vi "Init UI.vi"(8 "error in (no error)":errorcluster, 11 "Configuration Window in":refnum<class "Configuration Window.lvclass">) -> (0 "error out":errorcluster, 3 "Configuration Window out":refnum<class "Configuration Window.lvclass">)   [LabVIEW 2018, in "Configuration Window.lvlib" / "Configuration Window.lvclass"]
uses:
  Configuration Window.lvclass
  Configuration Window.lvclass/Configuration Window.ctl
  <userlib>/_OpenG.lib/file/file.llb/Strip Path Extension - 1D Array of Strings__ogtk.vi
  Main Panel/LF2R IDE/LF2R IDE.lvclass
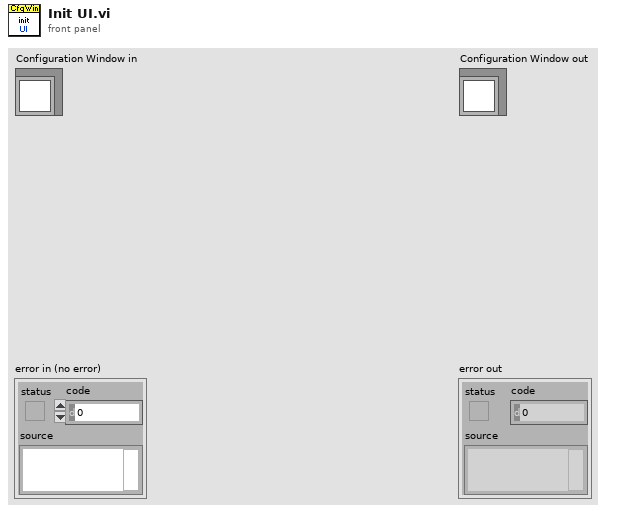
[diagram p1: front panel]
types:
  T1 = cluster{"Size":refnum<vi>, "Color":refnum<vi>, "Enable":refnum<vi>}
  T2 = cluster{"Fill Color":refnum<vi>, "Border Color":refnum<vi>, "Enable":refnum<vi>}
  T3 = cluster{"Fill Color":u32, "Border Color":u32, "Show?":bool}
  T4 = cluster{"_res_data":refnum<vi>, "_res_pngs":refnum<vi>}
  T5 = typedef "LF2R IDE.lvlib/LF2R IDE.lvclass/Const Path Setting.ctl" = cluster{"Data Folder Path":path, "PNG Folder Path":path}
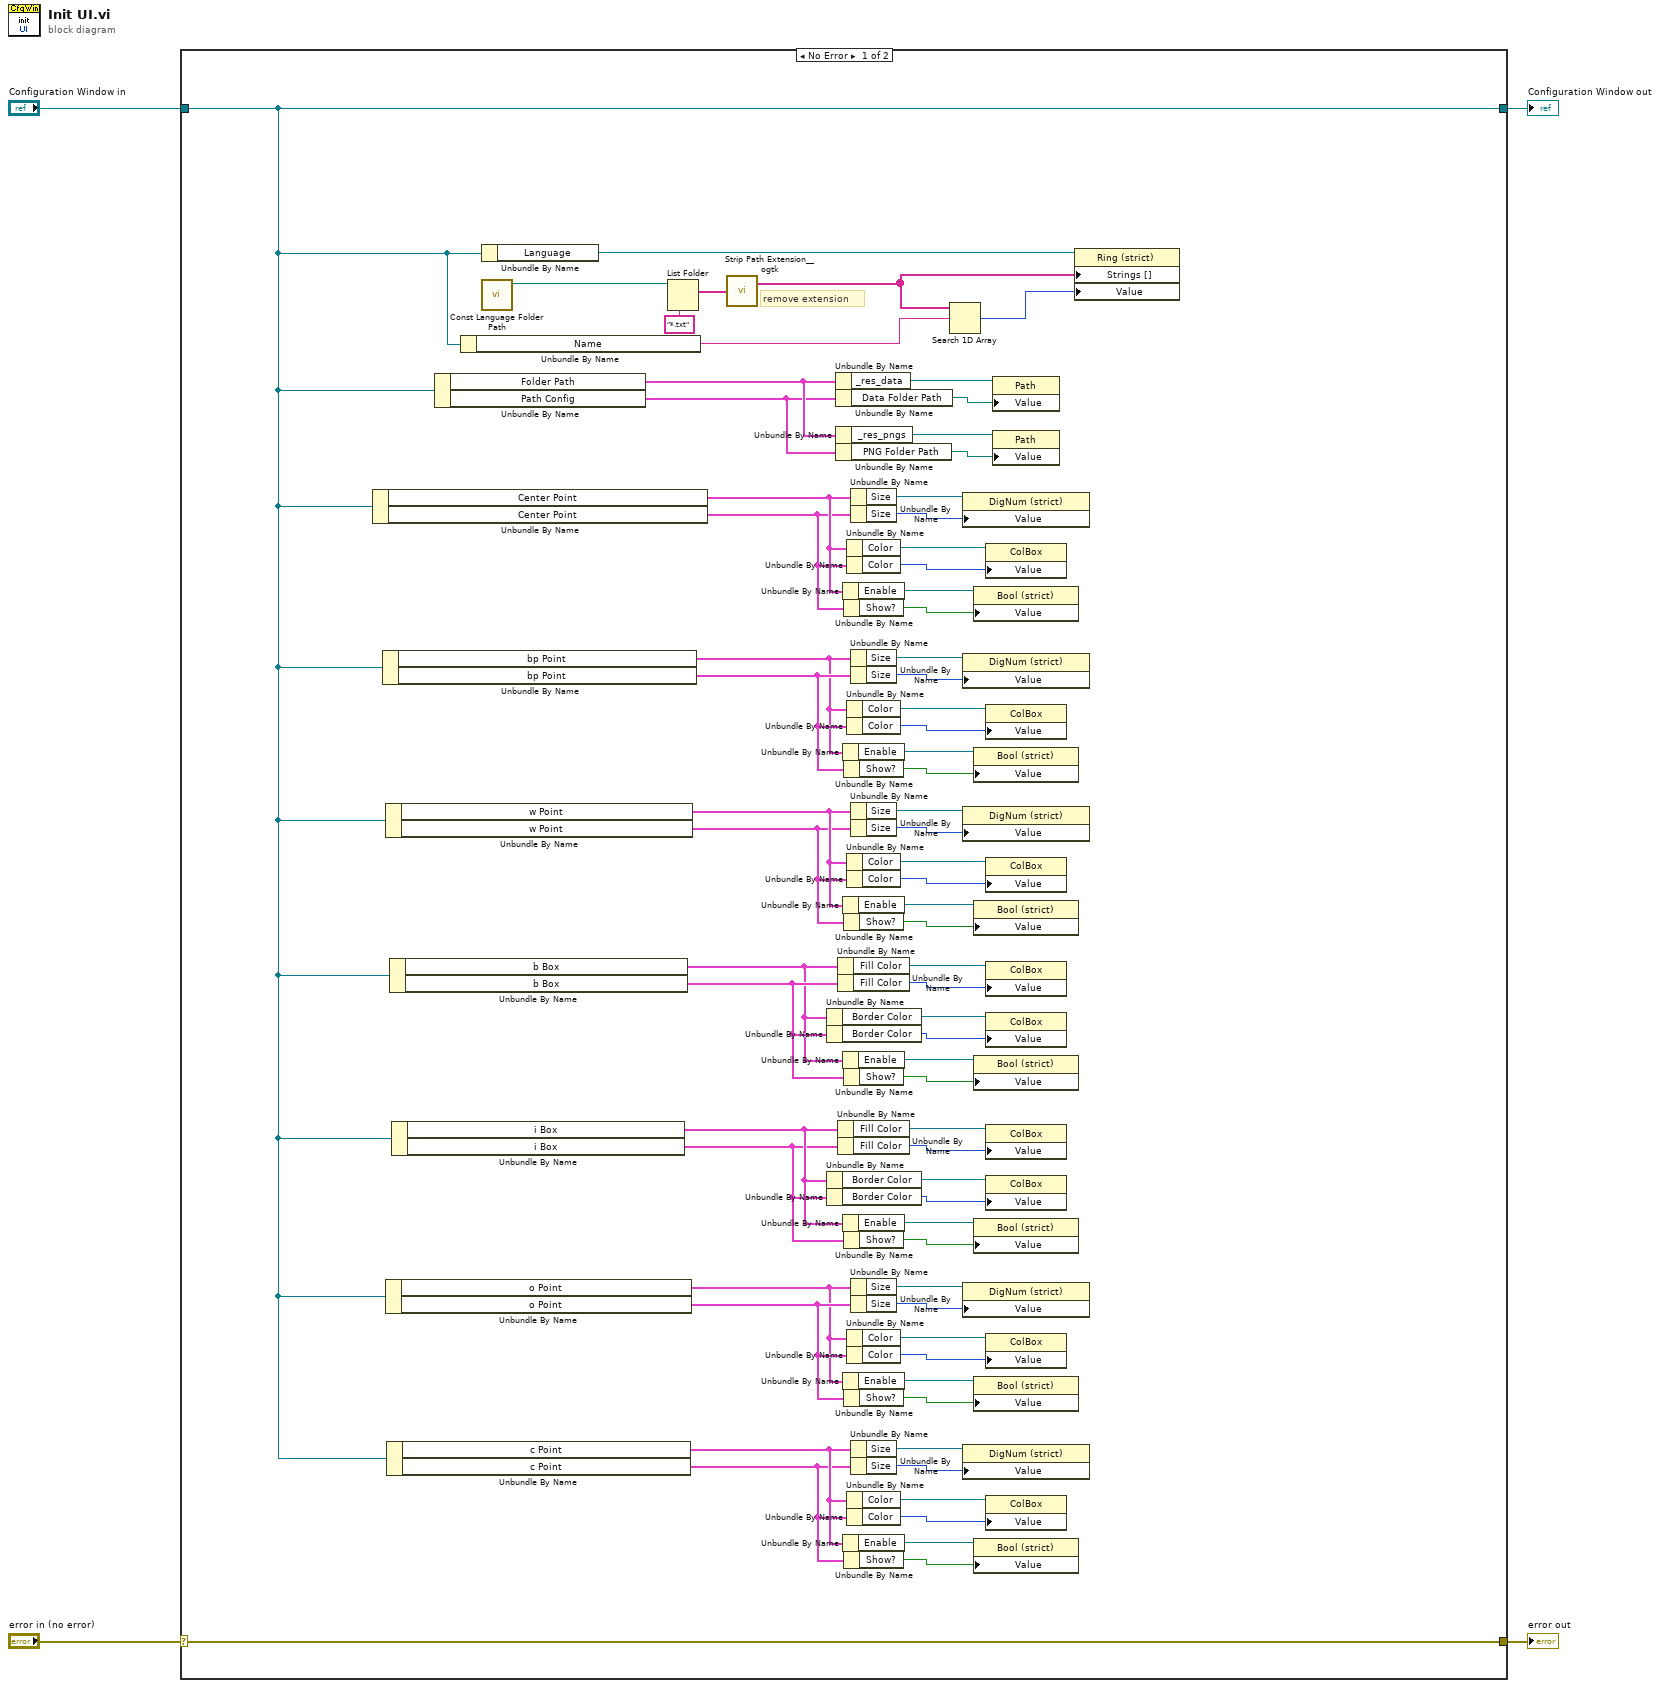
[diagram p0: block diagram]
diagram:
  n1 = case shown="No Error" "error in (no error)" {
    selector: "error in (no error)" -> [w75 w77]
    tunnel: [w75 w77] -> w3
    tunnel: [w6 w76] -> w1
    tunnel: "Configuration Window in" -> [w6 w76]
    frame No Error {
      # "remove extension"
      n2 = Unbundle By Name(w6) -> ("Center Point"=w62:T1, "Center Point"=w61:cluster{"Size":i32, "Color":u32, "Show?":bool})
      n3 = Unbundle By Name(w6) -> ("bp Point"=w59:T1, "bp Point"=w60:cluster{"Size":i32, "Color":u32, "Show?":bool})
      n4 = Unbundle By Name(w6) -> ("w Point"=w46:T1, "w Point"=w45:cluster{"Size":i32, "Color":u32, "Show?":bool})
      n5 = Unbundle By Name(w6) -> ("o Point"=w27:T1, "o Point"=w28:cluster{"Size":i32, "Color":u32, "Show?":bool})
      n6 = Unbundle By Name(w6) -> ("c Point"=w14:T1, "c Point"=w13:cluster{"Size":i32, "Color":u32, "Show?":bool})
      n7 = Unbundle By Name(w6) -> ("b Box"=w43:T2, "b Box"=w44:T3)
      n8 = Unbundle By Name(w6) -> ("i Box"=w30:T2, "i Box"=w29:T3)
      n9 = Unbundle By Name(w6) -> ("Folder Path"=w70:T4, "Path Config"=w69:T5)
      n10 = Unbundle By Name(w6) -> ("Name"=w5:string)
      n11 = Unbundle By Name(w6) -> ("Language"=w12:refnum<vi>)
      n12 = call "Const Language Folder Path.vi"() -> ("Language Folder Path"=w11:path)  [unwired: 11 in]
      n13 = List Folder(path=w11, pattern="*.txt") -> (filenames=w9:string[])  [unwired: 2 in, 3 out]
      n14 = call-poly <userlib>:"Strip Path Extension__ogtk.vi"("paths"=w9) -> ("roots"=w7:string[])  [unwired: 1 out]
      n15 = Unbundle By Name(w43) -> ("Border Color"=w40:refnum<vi>)
      n16 = Unbundle By Name(w44) -> ("Border Color"=w39:u32)
      n17 = Unbundle By Name(w30) -> ("Border Color"=w33:refnum<vi>)
      n18 = Unbundle By Name(w29) -> ("Border Color"=w34:u32)
      n19 = Unbundle By Name(w70) -> ("_res_data"=w74:refnum<vi>)
      n20 = Unbundle By Name(w69) -> ("Data Folder Path"=w73:path)
      n21 = Unbundle By Name(w70) -> ("_res_pngs"=w71:refnum<vi>)
      n22 = Unbundle By Name(w69) -> ("PNG Folder Path"=w72:path)
      n23 = Unbundle By Name(w43) -> ("Fill Color"=w37:refnum<vi>)
      n24 = Unbundle By Name(w44) -> ("Fill Color"=w38:u32)
      n25 = Unbundle By Name(w30) -> ("Fill Color"=w36:refnum<vi>)
      n26 = Unbundle By Name(w29) -> ("Fill Color"=w35:u32)
      n27 = Unbundle By Name(w62) -> ("Enable"=w64:refnum<vi>)
      n28 = Unbundle By Name(w59) -> ("Enable"=w57:refnum<vi>)
      n29 = Unbundle By Name(w46) -> ("Enable"=w48:refnum<vi>)
      n30 = Unbundle By Name(w43) -> ("Enable"=w41:refnum<vi>)
      n31 = Unbundle By Name(w30) -> ("Enable"=w32:refnum<vi>)
      n32 = Unbundle By Name(w27) -> ("Enable"=w25:refnum<vi>)
      n33 = Unbundle By Name(w14) -> ("Enable"=w16:refnum<vi>)
      n34 = Unbundle By Name(w61) -> ("Show?"=w63:bool)
      n35 = Unbundle By Name(w60) -> ("Show?"=w58:bool)
      n36 = Unbundle By Name(w45) -> ("Show?"=w47:bool)
      n37 = Unbundle By Name(w44) -> ("Show?"=w42:bool)
      n38 = Unbundle By Name(w29) -> ("Show?"=w31:bool)
      n39 = Unbundle By Name(w28) -> ("Show?"=w26:bool)
      n40 = Unbundle By Name(w13) -> ("Show?"=w15:bool)
      n41 = Unbundle By Name(w62) -> ("Color"=w65:refnum<vi>)
      n42 = Unbundle By Name(w61) -> ("Color"=w66:u32)
      n43 = Unbundle By Name(w59) -> ("Color"=w56:refnum<vi>)
      n44 = Unbundle By Name(w60) -> ("Color"=w55:u32)
      n45 = Unbundle By Name(w46) -> ("Color"=w49:refnum<vi>)
      n46 = Unbundle By Name(w45) -> ("Color"=w50:u32)
      n47 = Unbundle By Name(w27) -> ("Color"=w24:refnum<vi>)
      n48 = Unbundle By Name(w28) -> ("Color"=w23:u32)
      n49 = Unbundle By Name(w14) -> ("Color"=w17:refnum<vi>)
      n50 = Unbundle By Name(w13) -> ("Color"=w18:u32)
      n51 = Unbundle By Name(w62) -> ("Size"=w68:refnum<vi>)
      n52 = Unbundle By Name(w61) -> ("Size"=w67:i32)
      n53 = Unbundle By Name(w59) -> ("Size"=w53:refnum<vi>)
      n54 = Unbundle By Name(w60) -> ("Size"=w54:i32)
      n55 = Unbundle By Name(w46) -> ("Size"=w52:refnum<vi>)
      n56 = Unbundle By Name(w45) -> ("Size"=w51:i32)
      n57 = Unbundle By Name(w27) -> ("Size"=w21:refnum<vi>)
      n58 = Unbundle By Name(w28) -> ("Size"=w22:i32)
      n59 = Unbundle By Name(w14) -> ("Size"=w20:refnum<vi>)
      n60 = Unbundle By Name(w13) -> ("Size"=w19:i32)
      n61 = Search 1D Array(1D array=w7, element=w5) -> (index of element=w8:i32)  [unwired: 1 in]
      n62 = property class="DigNum (strict)"(reference=w68, "Value"=w67) -> ()  [unwired: 1 in, 2 out]
      n63 = property class="DigNum (strict)"(reference=w53, "Value"=w54) -> ()  [unwired: 1 in, 2 out]
      n64 = property class="DigNum (strict)"(reference=w52, "Value"=w51) -> ()  [unwired: 1 in, 2 out]
      n65 = property class="DigNum (strict)"(reference=w21, "Value"=w22) -> ()  [unwired: 1 in, 2 out]
      n66 = property class="DigNum (strict)"(reference=w20, "Value"=w19) -> ()  [unwired: 1 in, 2 out]
      n67 = property class="Bool (strict)"(reference=w64, "Value"=w63) -> ()  [unwired: 1 in, 2 out]
      n68 = property class="Bool (strict)"(reference=w57, "Value"=w58) -> ()  [unwired: 1 in, 2 out]
      n69 = property class="Bool (strict)"(reference=w48, "Value"=w47) -> ()  [unwired: 1 in, 2 out]
      n70 = property class="Bool (strict)"(reference=w41, "Value"=w42) -> ()  [unwired: 1 in, 2 out]
      n71 = property class="Bool (strict)"(reference=w32, "Value"=w31) -> ()  [unwired: 1 in, 2 out]
      n72 = property class="Bool (strict)"(reference=w25, "Value"=w26) -> ()  [unwired: 1 in, 2 out]
      n73 = property class="Bool (strict)"(reference=w16, "Value"=w15) -> ()  [unwired: 1 in, 2 out]
      n74 = property class="ColBox"(reference=w65, "Value"=w66) -> ()  [unwired: 1 in, 2 out]
      n75 = property class="ColBox"(reference=w56, "Value"=w55) -> ()  [unwired: 1 in, 2 out]
      n76 = property class="ColBox"(reference=w49, "Value"=w50) -> ()  [unwired: 1 in, 2 out]
      n77 = property class="ColBox"(reference=w37, "Value"=w38) -> ()  [unwired: 1 in, 2 out]
      n78 = property class="ColBox"(reference=w40, "Value"=w39) -> ()  [unwired: 1 in, 2 out]
      n79 = property class="ColBox"(reference=w36, "Value"=w35) -> ()  [unwired: 1 in, 2 out]
      n80 = property class="ColBox"(reference=w33, "Value"=w34) -> ()  [unwired: 1 in, 2 out]
      n81 = property class="ColBox"(reference=w24, "Value"=w23) -> ()  [unwired: 1 in, 2 out]
      n82 = property class="ColBox"(reference=w17, "Value"=w18) -> ()  [unwired: 1 in, 2 out]
      n83 = property class="Path"(reference=w74, "Value"=w73) -> ()  [unwired: 1 in, 2 out]
      n84 = property class="Path"(reference=w71, "Value"=w72) -> ()  [unwired: 1 in, 2 out]
      n85 = property class="Ring (strict)"(reference=w12, "Strings []"=w7, "Value"=w8) -> ()  [unwired: 1 in, 2 out]
    }
    frame Error {
    }
  }
  "error out" <- w3
  "Configuration Window out" <- w1
